vi "TimeDeliverStim.vi"() -> ()   [LabVIEW 2017]
uses:
  <vilib>/Analysis/baseanly.llb/Mean (DBL).vi
  <vilib>/DAQmx/write.llb/DAQmx Write.vi
  <vilib>/DAQmx/write.llb/DAQmx Write (Digital 1D Bool 1Chan 1Samp).vi
  <vilib>/DAQmx/configure/task.llb/DAQmx Start Task.vi
  <vilib>/DAQmx/configure/task.llb/DAQmx Wait Until Done.vi
  <vilib>/DAQmx/miscellaneous.llb/DAQmx Fill In Error Info.vi
  <vilib>/Analysis/NI_AALBase.lvlib
panel:
  out "Median run time (us)":dbl format="%0.2f"
  out "Mean run time (us)":dbl
  out "Histogram Graph":T1(graph)
  in  "n runs":i32=1000
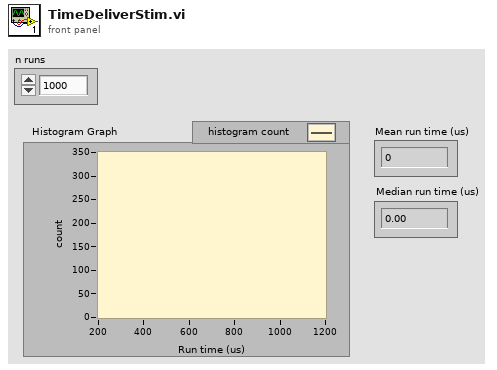
[diagram p1: front panel]
types:
  T1 = cluster{"X Values":dbl[], "Histogram: h(x)":i32[]}
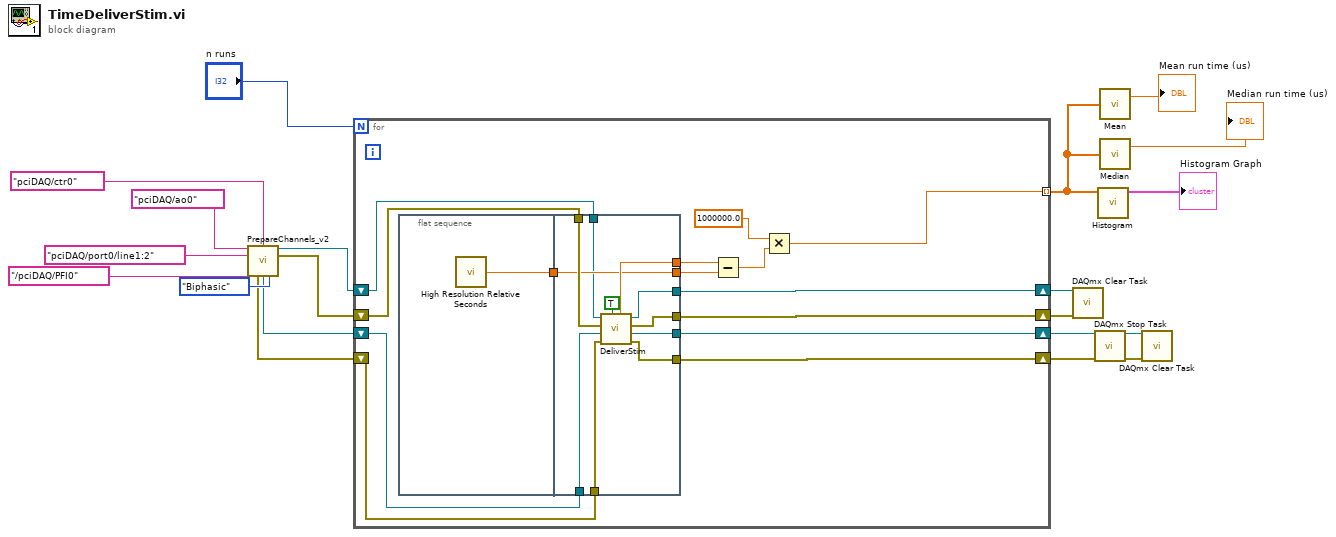
[diagram p0: block diagram]
diagram:
  n1 = call "PrepareChannels_v2.vi"("AO Physical channels"=tag "pciDAQ/ao0", "Onboard counter"=tag "pciDAQ/ctr0", "DO Physical channels"=tag "pciDAQ/port0/line1:2", "OEP sample clock in"=tag "/pciDAQ/PFI0", "Pulse Type"=enum16{"Monophasic", "Biphasic"}."Biphasic") -> ("AO task out"=w5:refnum<k21>, "AO error out"=w15:errorcluster, "DO error out"=w14:errorcluster, "DO task out"=w6:refnum<k21>)  [unwired: 4 in, 3 out]
  n2 = for {
    N: "n runs" -> [_]
    shift-right: [w26] -> w9
    shift-left: w15 -> [w33]
    shift-right: [w25] -> w8
    shift-left: w5 -> [w32]
    shift-right: [w28] -> w13
    shift-left: w14 -> [w31]
    shift-right: [w27] -> w12
    shift-left: w6 -> [w22]
    tunnel: [w21] -> w1 mode=indexing
    n3 = flat-sequence {
      tunnel: [w35] -> w34
      tunnel: w33 -> [w46]
      tunnel: w32 -> [w37]
      tunnel: w31 -> [w45]
      tunnel: w34 -> [w42]
      tunnel: [w43] -> w30
      tunnel: [w42] -> w29
      tunnel: [w41] -> w28
      tunnel: [w40] -> w27
      tunnel: [w39] -> w26
      tunnel: [w38] -> w25
      tunnel: w22 -> [w36]
      frame #0 {
        n4 = call <vilib>:"High Resolution Relative Seconds.vi"() -> ("relative seconds"=w35:dbl)
      }
      frame #1 {
        n5 = call "DeliverStim.vi"("Real stim on"=TRUE, "DO error in"=w45, "DO task in"=w36, "AO error in"=w46, "AO task in"=w37) -> ("DO error out"=w41:errorcluster, "DO task out"=w40:refnum<k21>, "AO error out"=w39:errorcluster, "AO task out"=w38:refnum<k21>, "Time done (s)"=w43:dbl)  [unwired: 1 in]
      }
    }
    n6 = Subtract(x=w30, y=w29) -> (x-y=w24:dbl)
    n7 = Multiply(x=1000000.0, y=w24) -> (x*y=w21:dbl)
  }
  n8 = call <vilib>:"DAQmx Clear Task.vi"("task in"=w8, "error in"=w9) -> ()  [unwired: 13 in, 1 out]
  n9 = call <vilib>:"DAQmx Stop Task.vi"("task/channels in"=w12, "error in"=w13) -> ("task out"=w11:refnum<k21>, "error out"=w10:errorcluster)  [unwired: 12 in]
  n10 = call <vilib>:"Histogram.vi"("X"=w1) -> ("Histogram Graph"=→"Histogram Graph":T1)  [unwired: 7 in, 3 out]
  n11 = call-poly <vilib>:"Mean.vi"("X"=w1) -> ("mean"=→"Mean run time (us)":dbl)  [unwired: 1 out]
  n12 = call <vilib>:"Median.vi"("X"=w1) -> ("median"=→"Median run time (us)":dbl)  [unwired: 1 out]
  n13 = call <vilib>:"DAQmx Clear Task.vi"("task in"=w11, "error in"=w10) -> ()  [unwired: 13 in, 1 out]
